vi "GetProxy.vi"(8 "error in (no error)":errorcluster, 11 "Subject in":refnum<class "Subject.lvclass">) -> (0 "error out":errorcluster, 3 "Proxy":refnum<class "Subject.lvclass">)   [LabVIEW 2014, in "forcible Proxy.lvlib" / "Subject.lvclass"]
uses:
  Subject.lvclass
  Proxy/OperationLogger (proxy).lvclass
  Proxy/OperationLogger (proxy).lvclass/OperationLogger (proxy).ctl
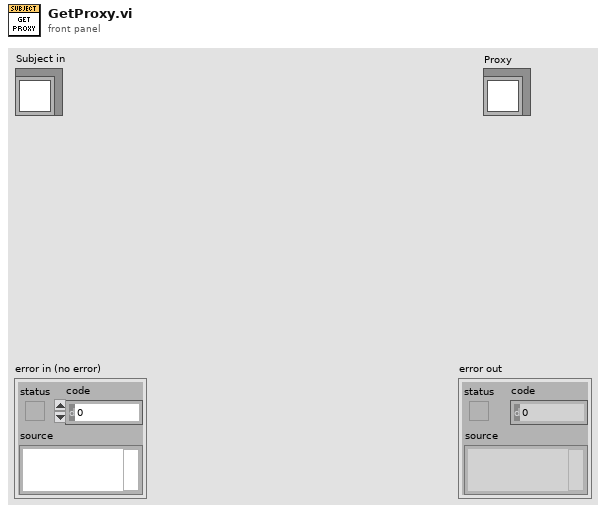
[diagram p1: front panel]
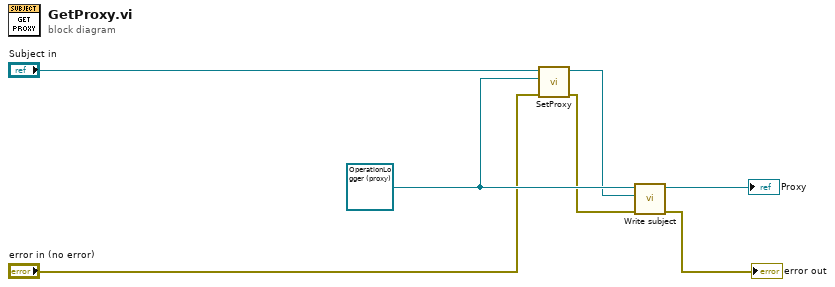
[diagram p0: block diagram]
diagram:
  w4 = refnum<class "OperationLogger (proxy).lvclass"> refnum ("forcible Proxy.lvlib:OperationLogger (proxy)")
  n1 = call "SetProxy.vi"("error in (no error)"="error in (no error)", "Proxy"=w4, "Subject in"="Subject in") -> ("error out"=w2:errorcluster, "Subject out"=w1:refnum<class "Subject.lvclass">)  [unwired: 7 in]
  n2 = call "Write subject.vi"("error in (no error)"=w2, "Normal Proxy.lvlib:Subject.lvclass"=w1, "OperationLogger (proxy) in"=w4) -> ("error out"=→"error out":errorcluster, "OperationLogger (proxy) out"=→"Proxy":refnum<class "OperationLogger (proxy).lvclass">)  [unwired: 7 in]
